vi "Start Reading.vi"(8 "error in (no error)":errorcluster, 10 "Baud Rate":u32=38400, 11 "COM Port":refnum<visa-resource-name>="COM4") -> (0 "error out":errorcluster, 1 "received str":string, 3 "Result":bool)   [LabVIEW 2018]
panel:
  # "START READING"
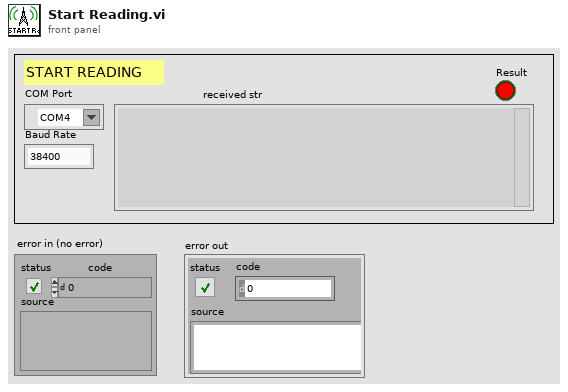
[diagram p1: front panel]
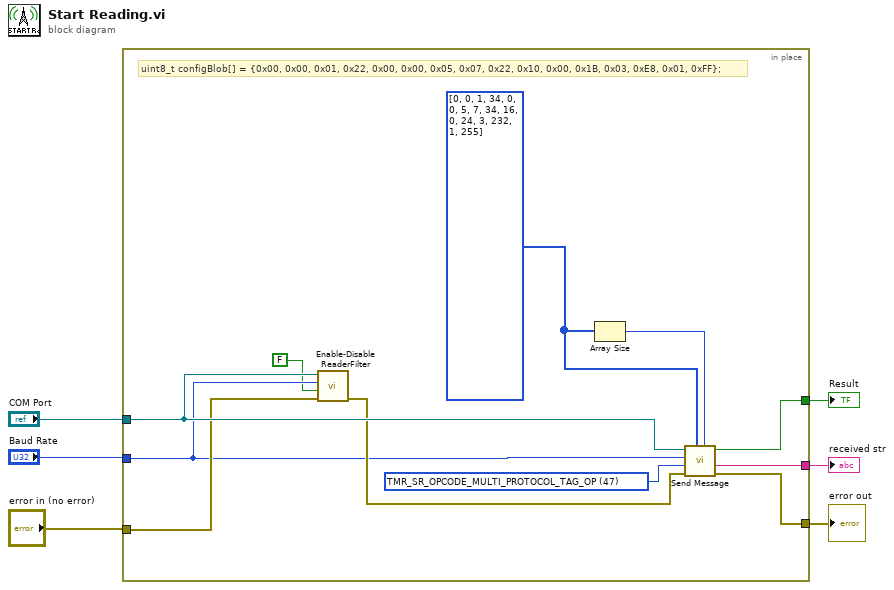
[diagram p0: block diagram]
diagram:
  n1 = in-place {
    in-place-border: "Baud Rate" -> [w8]
    in-place-border: "COM Port" -> [w11]
    in-place-border: "error in (no error)" -> [w10]
    in-place-border: [w15] -> w3
    in-place-border: [w17] -> w2
    in-place-border: [w16] -> w1
    w13 = u8[] [0, 0, 1, 34, 0, 0, 5, 7, 34, 16, 0, 24, 3, 232, 1, 255]
    w14 = u16 47 items=["TMR_SR_OPCODE_VERSION"=3, "TMR_SR_OPCODE_SET_BAUD_RATE"=6, "TMR_SR_OPCODE_READ_TAG_ID_SINGLE"=33, "TMR_SR_OPCODE_READ_TAG_ID_MULTIPLE"=34, "TMR_SR_OPCODE_WRITE_TAG_ID"=35, "TMR_SR_OPCODE_WRITE_TAG_DATA"=36, "TMR_SR_OPCODE_KILL_TAG"=38, "TMR_SR_OPCODE_READ_TAG_DATA"=40, "TMR_SR_OPCODE_CLEAR_TAG_ID_BUFFER"=42, "TMR_SR_OPCODE_MULTI_PROTOCOL_TAG_OP"=47, "TMR_SR_OPCODE_GET_READ_TX_POWER"=98, "TMR_SR_OPCODE_GET_WRITE_TX_POWER"=100, "TMR_SR_OPCODE_GET_POWER_MODE"=104, "TMR_SR_OPCODE_GET_READER_OPTIONAL_PARAMS"=106, "TMR_SR_OPCODE_GET_PROTOCOL_PARAM"=107, "TMR_SR_OPCODE_SET_ANTENNA_PORT"=145, "TMR_SR_OPCODE_SET_TAG_PROTOCOL"=147, "TMR_SR_OPCODE_SET_READ_TX_POWER"=146, "TMR_SR_OPCODE_SET_WRITE_TX_POWER"=148, "TMR_SR_OPCODE_SET_REGION"=151, "TMR_SR_OPCODE_SET_READER_OPTIONAL_PARAMS"=154, "TMR_SR_OPCODE_SET_PROTOCOL_PARAM"=155] ("Opcode Constant")
    # "uint8_t configBlob[] = {0x00, 0x00, 0x01, 0x22, 0x00, 0x00, 0x05, 0x07, 0x22, 0x10, 0x00, 0x1B, 0x03, 0xE8, 0x01, 0xFF};"
    n2 = call "Enable-Disable ReaderFilter.vi"("error in (no error)"=w10, "Enable/Disable"=FALSE, "Baud Rate"=w8, "COM Port"=w11) -> ("error out"=w9:errorcluster)  [unwired: 5 in, 2 out]
    n3 = Array Size(array=w13) -> (size(s)=w12:i32)
    n4 = call "Send Message.vi"("Size"=w12, "Data"=w13, "error in (no error)"=w9, "Opcode"=w14, "Baud Rate"=w8, "COM Port"=w11) -> ("error out"=w15:errorcluster, "received str"=w16:string, "Result"=w17:bool)  [unwired: 2 in, 1 out]
  }
  "error out" <- w3
  "Result" <- w2
  "received str" <- w1
